vi "Handle INVOCATION.vi"(8 "error in (no error)":errorcluster, 9 "Message Loop Shift Register Data":T1, 10 "Cluster":T16 {"Message Codes" items=["HELLO"=1, "WELCOME"=2, "ABORT"=3, "GOODBYE"=6, "ERROR"=8, "PUBLISH"=16, "PUBLISHED"=17, "SUBSCRIBE"=32, "SUBSCRIBED"=33, "UNSUBSCRIBE"=34, "UNSUBSCRIBED"=35, "EVENT"=36, "CALL"=48, "RESULT"=59, "REGISTER"=64, "REGISTERED"=65, "UNREGISTER"=66, "UNREGISTERED"=67, "INVOCATION"=68, "YIELD"=70]}, 11 "reference":refnum<class "WAMP Client.lvclass">) -> (0 "error out":errorcluster, 3 "reference out":refnum<class "WAMP Client.lvclass">)   [LabVIEW 2020, in "wamplv.lvlib" / "WAMP Client.lvclass"]
uses:
  WAMP Client.lvclass
  TypeDef/WAMP Received Message.ctl
  TypeDef/WAMP Message Codes.ctl
  TypeDef/Message Loop Shift Reg Data.ctl
  TypeDef/REGISTER Request Data.ctl
  TypeDef/Success or error.ctl
  API/TypeDefs/Combined error.ctl
  API/TypeDefs/WAMP error.ctl
  API/TypeDefs/INVOCATION payload.ctl
  TypeDef/Publish Requests Map.ctl
  TypeDef/PUBLISH Request Data.ctl
  TypeDef/PUBLISH result.ctl
  TypeDef/Endpoint Data.ctl
  TypeDef/CALL Request Map.ctl
  TypeDef/CALL Request Data.ctl
  API/TypeDefs/RESULT payload.ctl
  TypeDef/SUBSCRIBE Requests Map.ctl
  TypeDef/SUBSCRIBE Request Data.ctl
  TypeDef/Subscribe Result.ctl
  TypeDef/EVENT payload.ctl
  TypeDef/Subscriptions Map.ctl
  TypeDef/Subscription Details.ctl
  TypeDef/Unsubscribe Requests Map.ctl
  TypeDef/UNSUBSCRIBE Request Data.ctl
  TypeDef/UNSUBSCRIBE Result.ctl
  TypeDef/Unregister requests map.ctl
  TypeDef/Unregister request.ctl
  WAMP Client.lvclass/WAMP Client.ctl
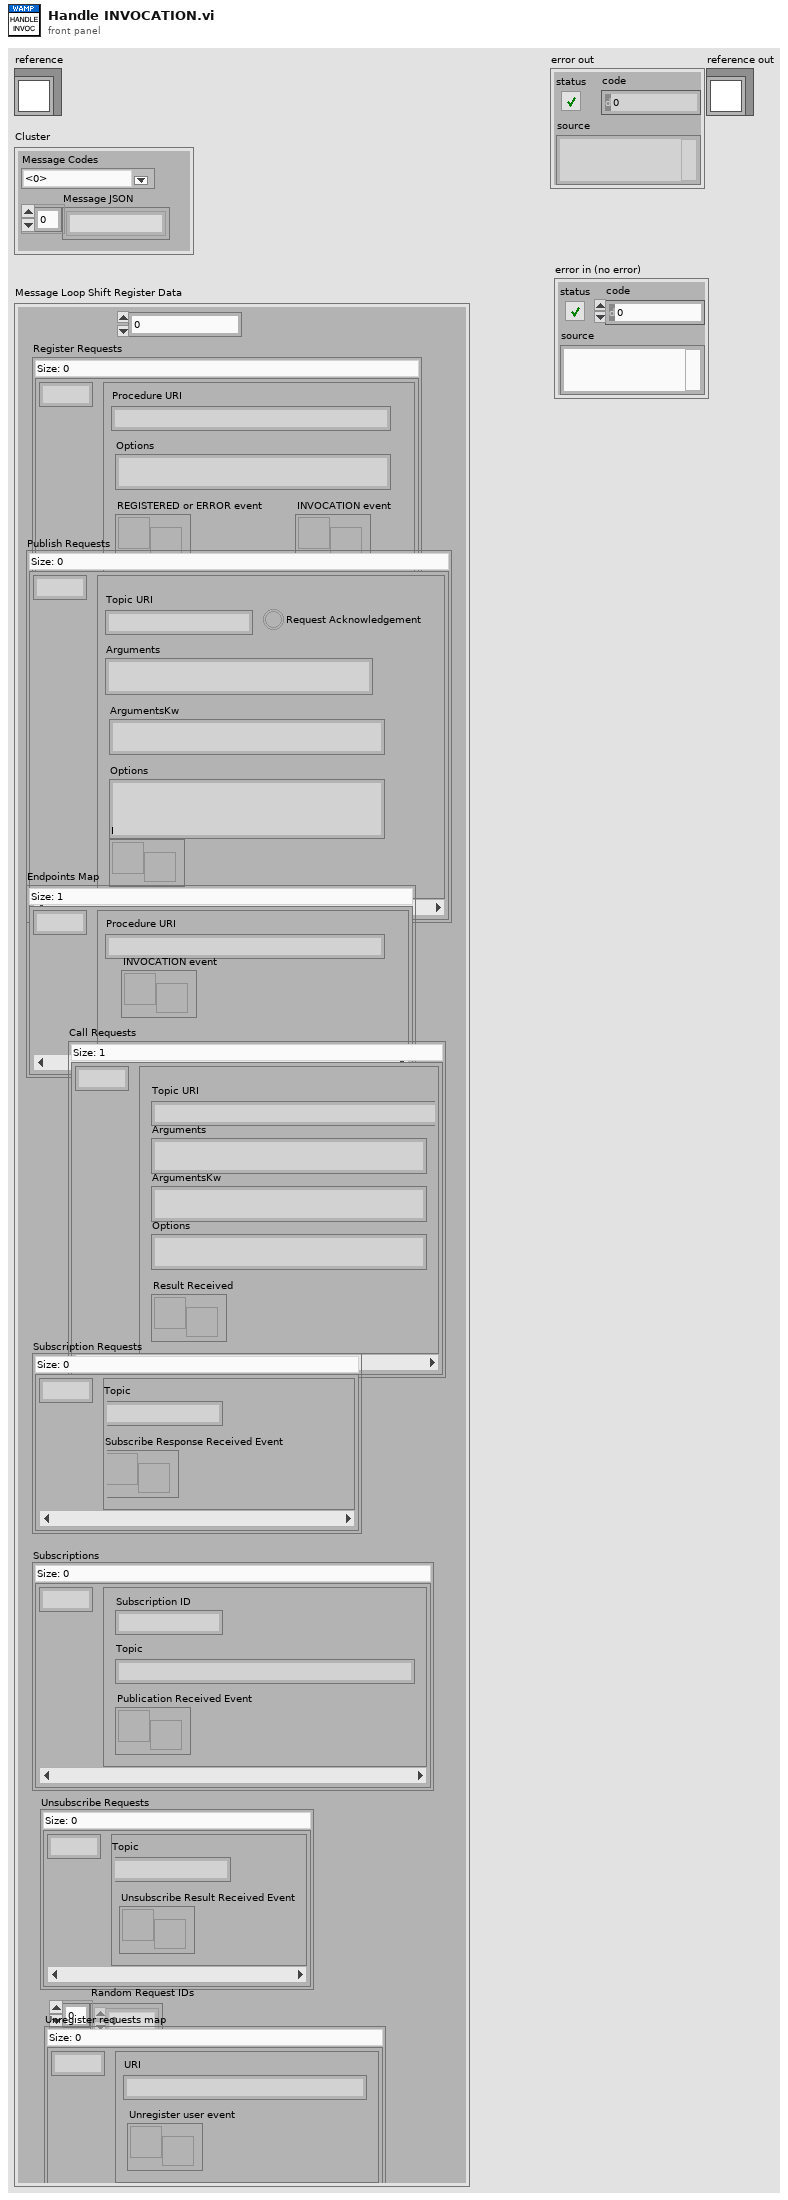
[diagram p1: front panel]
types:
  T1 = typedef "wamplv.lvlib/WAMP Client.lvclass/Message Loop Shift Reg Data.ctl" = cluster{"Last Request ID":u64, "Register Requests":map{u64, T2}, "Publish Requests":T3, "Endpoints Map":map{u64, T5}, "Call Requests":T6, "Subscription Requests":T8, "Subscriptions":T10, "Unsubscribe Requests":T12, "Random Request IDs":u64[], "Unregister requests map":T14}
  T2 = typedef "wamplv.lvlib/WAMP Client.lvclass/REGISTER Request Data.ctl" = cluster{"Procedure URI":string, "Options":string, "REGISTERED or ERROR event":refnum<user-event>, "INVOCATION event":refnum<user-event>}
  T3 = typedef "wamplv.lvlib/WAMP Client.lvclass/Publish Requests Map.ctl" = map{u64, T4}
  T4 = typedef "wamplv.lvlib/WAMP Client.lvclass/PUBLISH Request Data.ctl" = cluster{"Topic URI":string, "Arguments":string, "ArgumentsKw":string, "Publish Result Event":refnum<user-event>, "Request Acknowledgement":bool, "Options":string}
  T5 = typedef "wamplv.lvlib/WAMP Client.lvclass/Endpoint Data.ctl" = cluster{"Procedure URI":string, "INVOCATION event":refnum<user-event>}
  T6 = typedef "wamplv.lvlib/WAMP Client.lvclass/CALL Request Map.ctl" = map{u64, T7}
  T7 = typedef "wamplv.lvlib/WAMP Client.lvclass/CALL Request Data.ctl" = cluster{"Topic URI":string, "Arguments":string, "ArgumentsKw":string, "Result Received":refnum<user-event>, "Options":string}
  T8 = typedef "wamplv.lvlib/WAMP Client.lvclass/SUBSCRIBE Requests Map.ctl" = map{u64, T9}
  T9 = typedef "wamplv.lvlib/WAMP Client.lvclass/SUBSCRIBE Request Data.ctl" = cluster{"Topic":string, "Subscribe Response Received Event":refnum<user-event>}
  T10 = typedef "wamplv.lvlib/WAMP Client.lvclass/Subscriptions Map.ctl" = map{u64, T11}
  T11 = typedef "wamplv.lvlib/WAMP Client.lvclass/Subscription Details.ctl" = cluster{"Subscription ID":u64, "Topic":string, "Publication Received Event":refnum<user-event>}
  T12 = typedef "wamplv.lvlib/WAMP Client.lvclass/Unsubscribe Requests Map.ctl" = map{u64, T13}
  T13 = typedef "wamplv.lvlib/WAMP Client.lvclass/UNSUBSCRIBE Request Data.ctl" = cluster{"Topic":string, "Unsubscribe Result Received Event":refnum<user-event>}
  T14 = typedef "wamplv.lvlib/WAMP Client.lvclass/Unregister requests map.ctl" = map{u64, T15}
  T15 = typedef "wamplv.lvlib/WAMP Client.lvclass/Unregister request.ctl" = cluster{"URI":string, "Unregister user event":refnum<user-event>}
  T16 = typedef "wamplv.lvlib/WAMP Client.lvclass/WAMP Received Message.ctl" = cluster{"Message JSON":string[], "Message Codes":T17}
  T17 = typedef "wamplv.lvlib/WAMP Client.lvclass/WAMP Message Codes.ctl" = u16
  T18 = typedef "wamplv.lvlib/WAMP Client.lvclass/INVOCATION payload.ctl" = cluster{"Arguments":string, "ArgumentKw":string, "Procedure URI":string, "Details":string, "Registration ID":u64, "Request ID":u64}
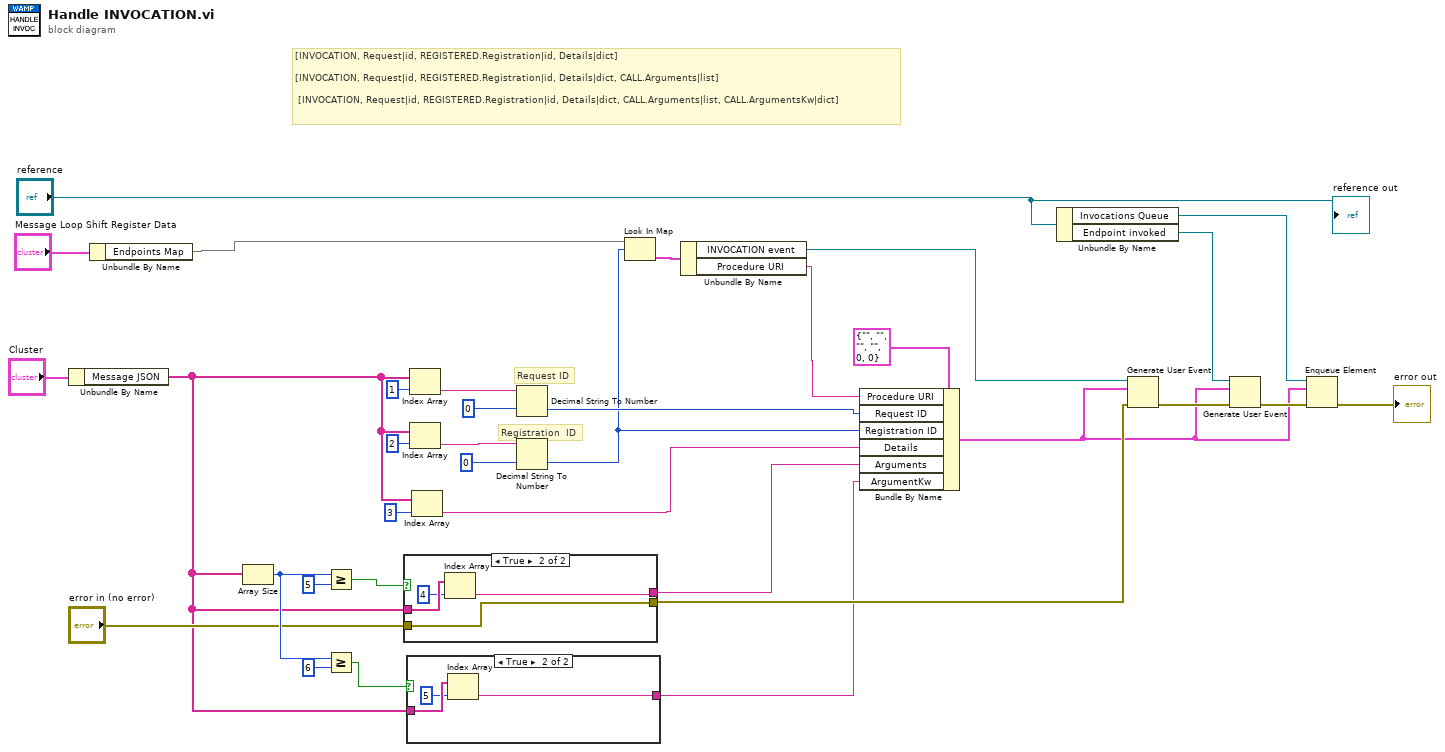
[diagram p0: block diagram]
diagram:
  # "[INVOCATION, Request|id, REGISTERED.Registration|id, Details|dict]\n\n[INVOCATION, Request|id, REGISTERED.Registration|id, Details|dict, CALL.Arguments|list]\n\n [INVOCATION, Request|id, REGISTERED.Registration|id, Details|dict, CALL.Arguments|list, CALL.ArgumentsKw|dict]"
  # "Registration  ID"
  # "Request ID"
  n1 = Unbundle By Name("Cluster") -> ("Message JSON"=w7:string[])
  n2 = Unbundle By Name("Message Loop Shift Register Data") -> ("Endpoints Map"=w13:map{u64, T5})
  n3 = Array Size(array=w7) -> (size(s)=w24:i32)
  n4 = Greater Or Equal?(x=w24, y=5) -> (x >= y?=w26:bool)
  n5 = Greater Or Equal?(x=w24, y=6) -> (x >= y?=w23:bool)
  n6 = case shown="True" w26 {
    tunnel: w7 -> [_ w39]
    tunnel: [_ w36] -> w9
    tunnel: "error in (no error)" -> [w35 w37]
    tunnel: [w35 w37] -> w21
    frame False {
    }
    frame True {
      n7 = Index Array(array=w39, index=4) -> (element=w36:string)
    }
  }
  n8 = case shown="True" w23 {
    tunnel: w7 -> [_ w42]
    tunnel: [_ w40] -> w8
    frame False {
    }
    frame True {
      n9 = Index Array(array=w42, index=5) -> (element=w40:string)
    }
  }
  n10 = Index Array(array=w7, index=1) -> (element=w33:string)
  n11 = Index Array(array=w7, index=2) -> (element=w34:string)
  n12 = Index Array(array=w7, index=3) -> (element=w10:string)
  n13 = Decimal String To Number(string=w33, default (0L)=u64 0) -> (number=w12:u64)  [unwired: 1 in, 1 out]
  n14 = Decimal String To Number(string=w34, default (0L)=u64 0) -> (number=w11:u64)  [unwired: 1 in, 1 out]
  n15 = Look In Map(map=w13, key=w11) -> (value=w19:T5)  [unwired: 1 in, 1 out]
  n16 = Unbundle By Name(w19) -> ("INVOCATION event"=w5:refnum<user-event>, "Procedure URI"=w18:string)
  n17 = Bundle By Name(cluster=T18 {"Arguments"="", "ArgumentKw"="", "Procedure URI"="", "Details"="", "Registration ID"=0, "Request ID"=0} ("INVOCATION payload"), "Procedure URI"=w18, "Request ID"=w12, "Registration ID"=w11, "Details"=w10, "Arguments"=w9, "ArgumentKw"=w8) -> (w1:T18)
  n18 = Unbundle By Name("reference") -> ("Invocations Queue"=w2:refnum<queue>, "Endpoint invoked"=w16:refnum<user-event>)
  n19 = Generate User Event(user event=w5, event data cluster=w1, error in=w21) -> (error out=w15:errorcluster)  [unwired: 1 in, 1 out]
  n20 = Generate User Event(user event=w16, event data cluster=w1, error in=w15) -> (error out=w4:errorcluster)  [unwired: 1 in, 1 out]
  n21 = Enqueue Element(queue=w2, element=w1, error in (no error)=w4) -> (error out=→"error out":errorcluster)  [unwired: 1 in, 2 out]
  "reference out" <- "reference"
